vi "Configure Frequency Sweep.vi"(7 "Steps Value (0)":i32, 8 "error in (no error)":errorcluster, 9 "Stop Frequency (5E+7 Hz)":dbl=50000000.0, 10 "Start Frequency (5E+7 Hz)":dbl=50000000.0, 11 "VISA resource name":refnum<visa-resource-name>) -> (0 "error out":errorcluster, 3 "VISA resource name out":refnum<visa-resource-name>)   [LabVIEW 2018, in "Agilent U2000 Series.lvlib"]
doc: "Sets the start, stop, step frequency for frequency sweep.\n\nNote: \nThis VI is only applicable for U2040 X-Series."
uses:
  Agilent U2000 Series.lvlib
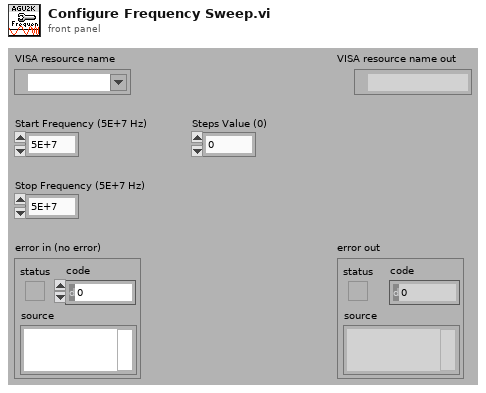
[diagram p1: front panel]
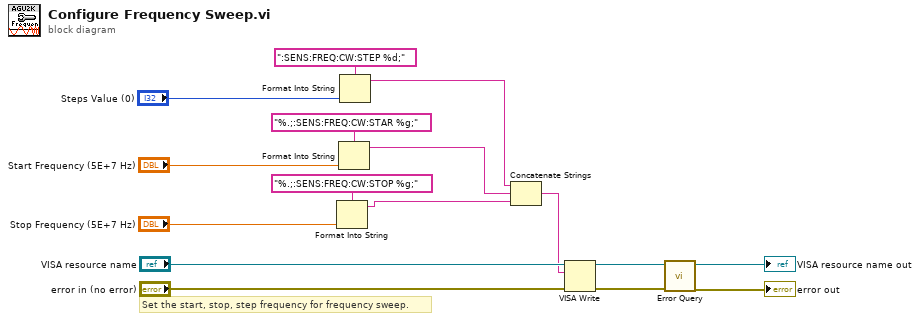
[diagram p0: block diagram]
diagram:
  # "Set the start, stop, step frequency for frequency sweep."
  n1 = Format Into String(format string="%.;:SENS:FREQ:CW:STOP %g;", "Stop Frequency (5E+7 Hz)") -> (resulting string=w4:string)  [unwired: 2 in, 1 out]
  n2 = Format Into String(format string="%.;:SENS:FREQ:CW:STAR %g;", "Start Frequency (5E+7 Hz)") -> (resulting string=w3:string)  [unwired: 2 in, 1 out]
  n3 = Format Into String(format string=":SENS:FREQ:CW:STEP %d;", "Steps Value (0)") -> (resulting string=w2:string)  [unwired: 2 in, 1 out]
  n4 = Concatenate Strings(w2, w3, w4) -> (w1:string)
  n5 = VISA Write(VISA resource name="VISA resource name", write buffer=w1, error in (no error)="error in (no error)") -> (VISA resource name out=w8:refnum<visa-resource-name>, error out=w7:errorcluster)  [unwired: 1 out]
  n6 = call "Error Query.vi"("error in (no error)"=w7, "VISA resource name"=w8) -> ("error out"=→"error out":errorcluster, "VISA resource name out"=→"VISA resource name out":refnum<visa-resource-name>)  [unwired: 6 in, 2 out]
